vi "List and Apply SystemLink State.vi"() -> ()   [LabVIEW 2017]
doc: "This example shows how to open a connection to the SystemLink server and get a list of states."
uses:
  SystemLink_States_API.lvlib
panel:
  out "List of State IDs":string[](array[string])
  in  "password":string
  in  "username":string
  in  "SystemLink server base URL":string="https://"
  out "List of State Names":string[](array[string])
  # "SystemLink Server"
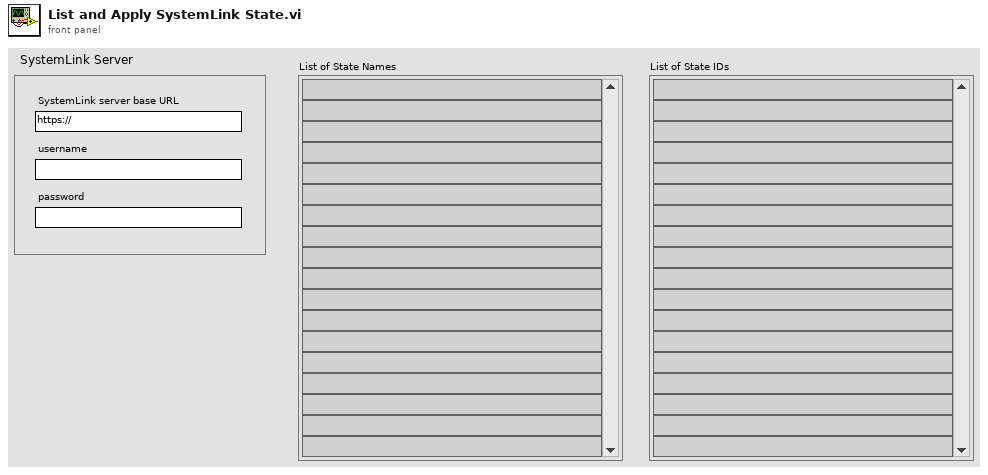
[diagram p1: front panel]
types:
  T1 = typedef "SystemLink_States_API.lvlib/systemlink repo.ctl" = cluster{"client handle out":T2, "SystemLink server base URL":string}
  T2 = typedef "LabVIEWHTTPClient.lvlib/ClientHandle.ctl" = refnum<k1>
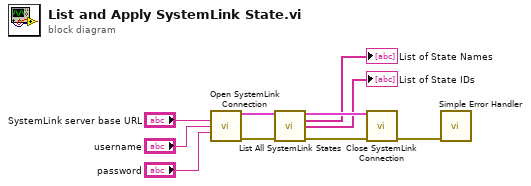
[diagram p0: block diagram]
diagram:
  n1 = call "Open SystemLink Connection.vi"("SystemLink server base URL"="SystemLink server base URL", "username"="username", "password"="password") -> ("SystemLink connection out"=w6:T1, "error out"=w4:errorcluster)  [unwired: 11 in]
  n2 = call "List All SystemLink States.vi"("SystemLink connection in"=w6, "error in (no error)"=w4) -> ("SystemLink connection out"=w5:T1, "SystemLink State Names"=→"List of State Names":string[], "SystemLink State IDs"=→"List of State IDs":string[], "error out"=w3:errorcluster)  [unwired: 10 in]
  n3 = call "Close SystemLink Connection.vi"("SystemLink connection in"=w5, "error in (no error)"=w3) -> ("error out"=w7:errorcluster)  [unwired: 13 in]
  n4 = call <vilib>:"Simple Error Handler.vi"("error in (no error)"=w7) -> ()  [unwired: 4 in, 5 out]
